vi "DockerTools - Update application.vi"(8 "Error In":errorcluster) -> (0 "Error Out":errorcluster)   [LabVIEW 2017]
panel:
  out "Firefly iii App Container ID":string
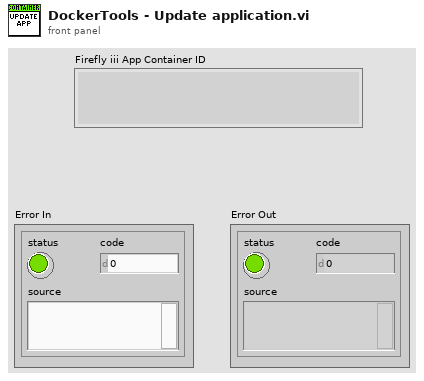
[diagram p1: front panel]
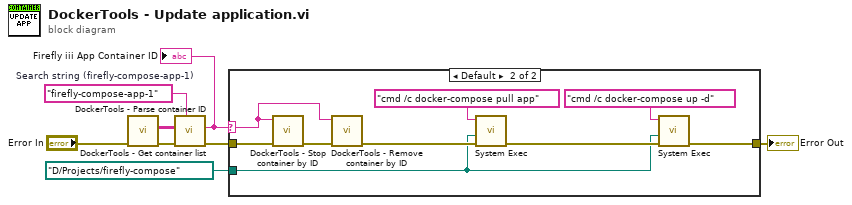
[diagram p0: block diagram]
diagram:
  w2 = "firefly-compose-app-1"  # Search string (firefly-compose-app-1)
  n1 = call "DockerTools - Get container list.vi"("error in"="Error In") -> ("error out"=w8:errorcluster, "Container list"=w1:string[][])  [unwired: 8 in, 1 out]
  n2 = call "DockerTools - Parse container ID.vi"("String (firefly-compose-app-1)"=w2, "Error In"=w8, "Container list"=w1) -> ("Error Out"=w6:errorcluster, "Firefly iii App Container ID"=w3:string)  [unwired: 7 in]
  "Firefly iii App Container ID" <- w3
  n3 = case shown="Default" w3 {
    selector: w3 -> [_ w10]
    tunnel: w6 -> [w9 w18]
    tunnel: [w9 w17] -> w5
    tunnel: path "D:/Projects/firefly-compose" ("working directory") -> [_ w11]
    frame "" {
    }
    frame Default {
      n4 = call "DockerTools - Stop container by ID.vi"("error in"=w18, "Container ID"=w10) -> ("error out"=w15:errorcluster)  [unwired: 9 in]
      n5 = call "DockerTools - Remove container by ID.vi"("error in"=w15, "String"=w10) -> ("error out"=w14:errorcluster)  [unwired: 9 in]
      n6 = call <vilib>:"System Exec.vi"("error in (no error)"=w14, "working directory"=w11, "command line"="cmd /c docker-compose pull app") -> ("error out"=w13:errorcluster)  [unwired: 5 in, 3 out]
      n7 = call <vilib>:"System Exec.vi"("error in (no error)"=w13, "working directory"=w11, "command line"="cmd /c docker-compose up -d") -> ("error out"=w17:errorcluster)  [unwired: 5 in, 3 out]
    }
  }
  "Error Out" <- w5
